vi "ProbeStationAutomation.vi"() -> ()   [LabVIEW 2020]
uses:
  Control 2.ctl
  C:/Users/User/Desktop/Automation/CurrentVersion/LabviewDXFViewer/bin/Release/LabviewDXFViewer.exe
  LabviewDXFViewer/bin/Release/LabviewDXFViewer.exe
  UIReferences.ctl
  WaferAlignmentType.ctl
  <vilib>/Utility/file.llb/Write Delimited Spreadsheet (DBL).vi
  Keithley 2600 Series/Keithley 2600 Series.lvlib
panel:
  in  "StartOxide":refnum<k24>(container)
  out "WaferAlignment":T1
  out "UiDefinition 3":T2
  in  "PathInfos":T3
  in  "UiDefinition 2":T2
  out "SweepInfo":T4
  out "error out":errorcluster
  out "Position 3":i32[](array[numeric])
  out "Position 2":i32[](array[numeric])
  out "Status":string="Please Load/Select probe site list"
  in  "Chip Orientation":i32(ring) items=["Horizontal", "Vertical"]
  in  "TextEditor":refnum<k24>(container)
  out "WaferTestPoints":string
  out "TestPointsLoaded":bool
  out "dxfFile":string
  out "error out 5":errorcluster
  out "Fit Array":string[][](array[string])
  out "error out 4":errorcluster
  out "error out 3":errorcluster
  out "Fit":dbl[][](array[numeric])
  out "IV Scan Data":dbl[][](array[numeric])
  out "Rotation Misalign":dbl[](array[numeric])
  out "Scale Misalign":dbl
  out "Position 1":i32[](array[numeric])
  in  "Microsites":refnum<k24>(container)
  in  "DXFCanvas":refnum<k24>(container)
  in  "WebCamViewer":refnum<k24>(container)
  in  "IV Curves":T5
  in  "Tab Control":T6(tab)
  in  "ClearPositions":bool
  in  "User":string
  in  "resetcontact":bool
  in  "EnableJoystick":bool
  in  "StartCycle":refnum<k24>(container)
  in  "Version":string
  in  "Experiment":string
  in  "Lower":refnum<k24>(container)
  in  "Raise":refnum<k24>(container)
  in  "West":refnum<k24>(container)
  in  "East":refnum<k24>(container)
  in  "North":refnum<k24>(container)
  in  "South":refnum<k24>(container)
  in  "Align Position 1":bool
  in  "Platten Move":refnum<k24>(container)
  in  "Masks":string(combo)
  in  "Move Position 1":bool
  in  "Align Position 3":bool
  in  "Position 3":bool
  in  "Align Position 2":bool
  in  "Position 2":bool
  in  "Die":string
  in  "Wafer":string
  in  "Jog (um) 2":dbl=100.0
  in  "Jog (um)":dbl=500.0
  in  "Load Mask":bool
  in  "Save Wafer":bool
  in  "Lift Distance (um)":dbl=2000.0
  in  "Quit":bool
  out "In Contact":bool
  out "Motor Position":string
  in  "Save Tag":string
  out "Capacitance":dbl
  in  "Current Range (A)":dbl=1e-10
  in  "Junction":string(combo)="None"
  in  "Sweeps":dbl=2.0
  in  "Number Points":dbl=200.0
  in  "Minimum (mV)":dbl=-100.0
  in  "Maxiumum (mV)":dbl=100.0
  in  "Source Measure Unit Channel (0: Channel A)":i32(ring) items=["Channel A", "Channel B"]
  in  "VISA resource name":refnum<visa-resource-name>="Keithley_2636A"
  in  "Scan":bool
  in  "Save Scan":bool
  out "Conductance":dbl
  out "Intercept":dbl
  out "XY Graph":cluster{"x":timestamp, "y":dbl}[](graph)
  in  "Steps Per micron":dbl=0.629
  in  "Stepper Controller Port":i32=3
  out "GetCameras":string[](array[string])
  in  "Wafer Definition File":path=path "C:/Users/User/Desktop/Automation/ASU FG Mask 21.08.26.dxf"
  in  "Wafer Units to microns":dbl=1.0
  in  "Data Path":path=path "C:/Data"
  # "Run Oxide"
  # "Optional Tags"
  # "Jog Platten"
  # "Platten Altitude"
  # "Run IVs"
  # "Cycle Step"
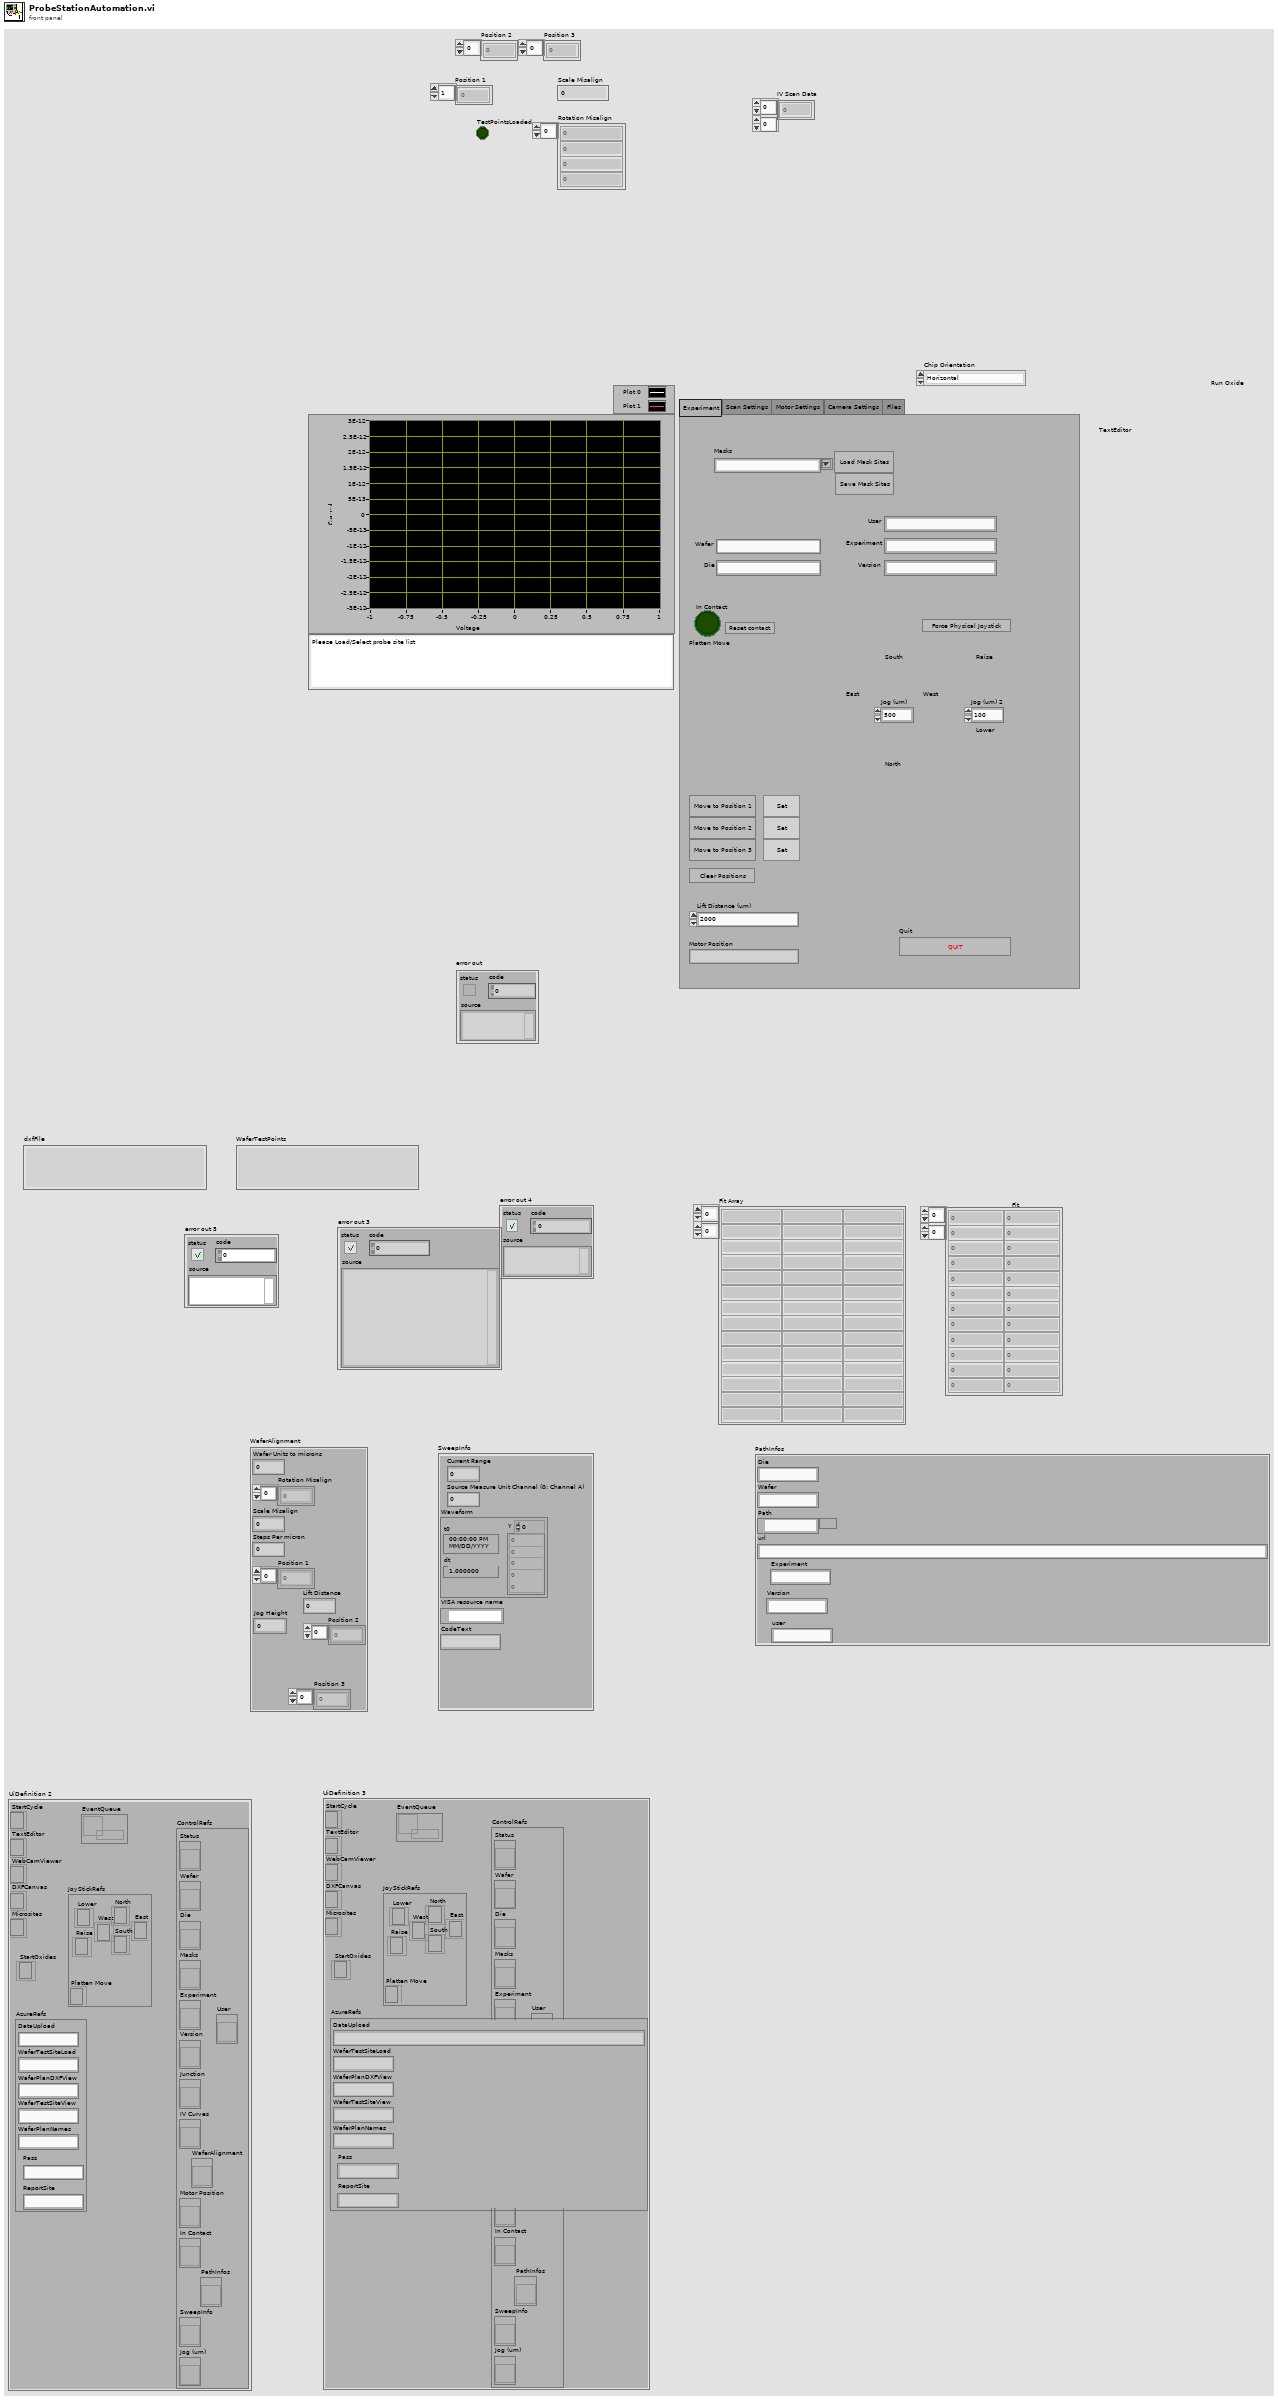
[diagram p1: front panel]
types:
  T1 = typedef "WaferAlignmentType.ctl" = cluster{"Wafer Units to microns":dbl, "Rotation Misalign":dbl[], "Scale Misalign":dbl, "Steps Per micron":dbl, "Position 1":i32[], "Position 2":i32[], "Lift Distance":i32, "Position 3":i32[], "Jog Height":i32}
  T2 = typedef "UIReferences.ctl" = cluster{"StartCycle":refnum<k24>, "TextEditor":refnum<k24>, "WebCamViewer":refnum<k24>, "DXFCanvas":refnum<k24>, "Microsites":refnum<k24>, "JoyStickRefs":cluster{"North":refnum<k24>, "Lower":refnum<k24>, "Raise":refnum<k24>, "Platten Move":refnum<k24>, "West":refnum<k24>, "East":refnum<k24>, "South":refnum<k24>}, "AzureRefs":cluster{"DataUpload":string, "WaferTestSiteLoad":string, "WaferPlanDXFView":string, "WaferTestSiteView":string, "WaferPlanNames":string, "Pass":string, "ReportSite":string}, "ControlRefs":cluster{"Status":refnum<vi>, "Wafer":refnum<vi>, "Die":refnum<vi>, "Masks":refnum<vi>, "Experiment":refnum<vi>, "Version":refnum<vi>, "Junction":refnum<vi>, "IV Curves":refnum<vi>, "Motor Position":refnum<vi>, "In Contact":refnum<vi>, "SweepInfo":refnum<vi>, "Jog (um)":refnum<vi>, "PathInfos":refnum<vi>, "User":refnum<vi>, "WaferAlignment":refnum<vi>}, "EventQueue":refnum<queue>, "StartOxides":refnum<k24>}
  T3 = cluster{"Die":string, "Wafer":string, "Path":path, "url":string, "Experiment":string, "Version":string, "user":string}
  T4 = cluster{"Current Range":dbl, "Source Measure Unit Channel (0: Channel A)":i32, "Waveform":waveform(dbl), "VISA resource name":refnum<visa-resource-name>, "CodeText":string}
  T5 = typedef "Control 2.ctl" = cluster{"Y":dbl[], "Current (A)":dbl[]}
  T6 = enum32{"Experiment", "Scan Settings", "Motor Settings", "Camera Settings", "Files"}
  T7 = cluster{"DataUpload":string, "WaferTestSiteLoad":string, "WaferPlanDXFView":string, "WaferTestSiteView":string, "WaferPlanNames":string, "Pass":string, "ReportSite":string}
  T8 = cluster{"North":refnum<k24>, "Lower":refnum<k24>, "Raise":refnum<k24>, "Platten Move":refnum<k24>, "West":refnum<k24>, "East":refnum<k24>, "South":refnum<k24>}
  T9 = cluster{"Status":refnum<vi>, "Wafer":refnum<vi>, "Die":refnum<vi>, "Masks":refnum<vi>, "Experiment":refnum<vi>, "Version":refnum<vi>, "Junction":refnum<vi>, "IV Curves":refnum<vi>, "Motor Position":refnum<vi>, "In Contact":refnum<vi>, "SweepInfo":refnum<vi>, "Jog (um)":refnum<vi>, "PathInfos":refnum<vi>, "User":refnum<vi>, "WaferAlignment":refnum<vi>}
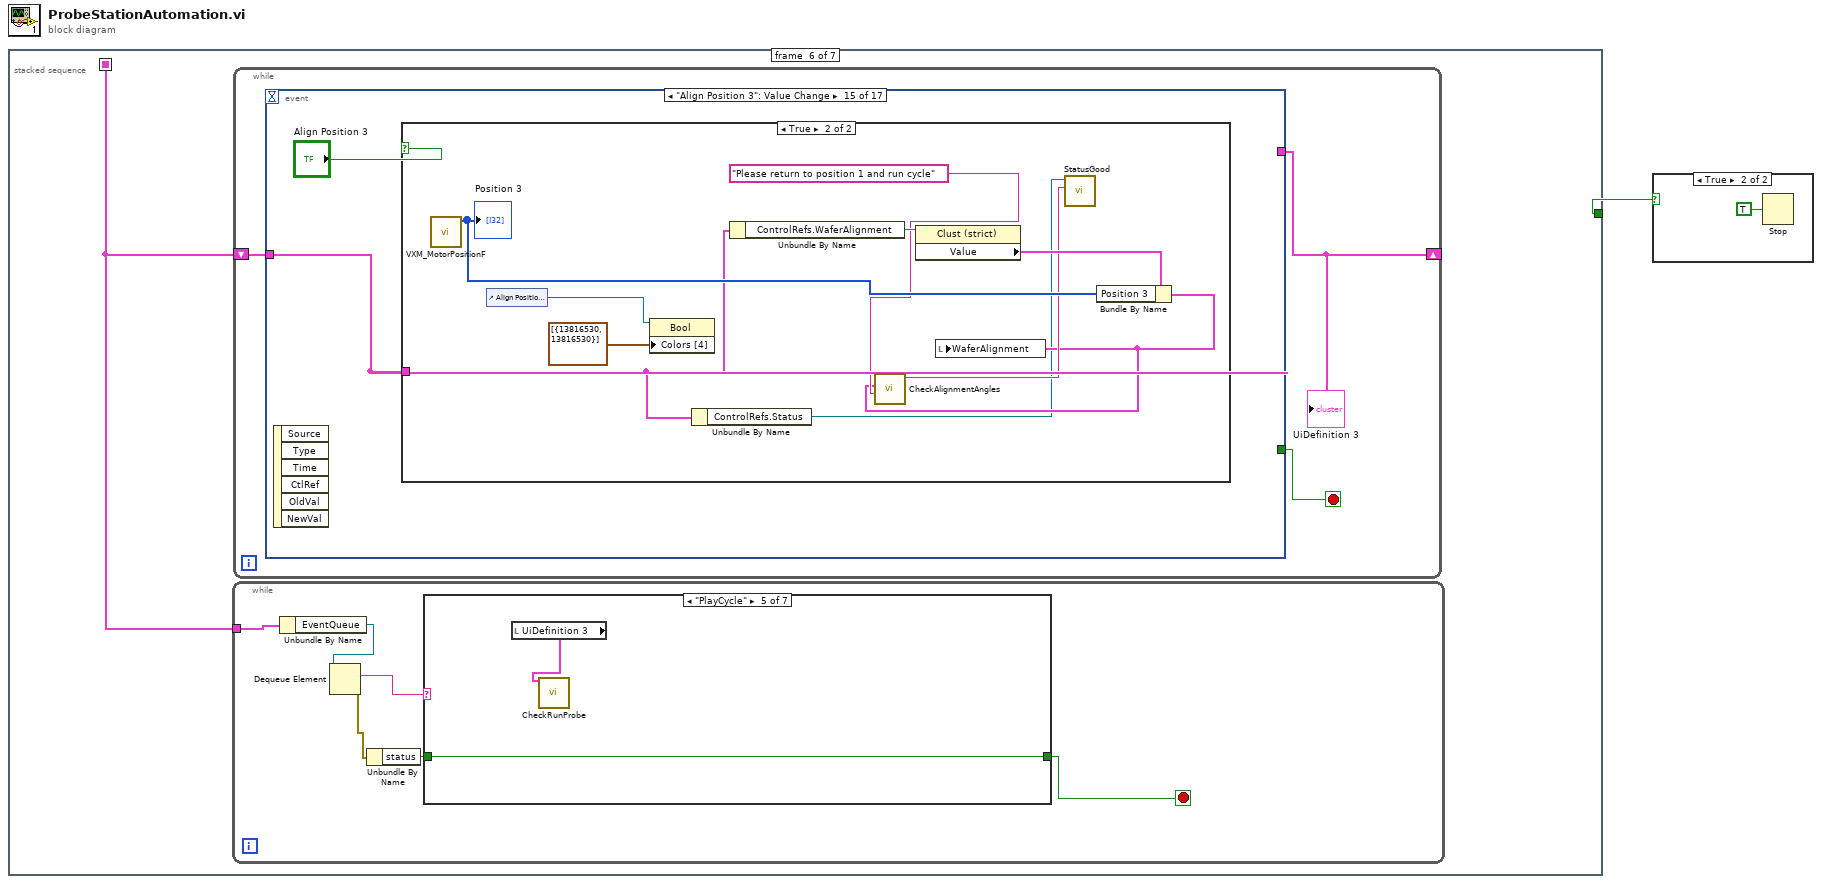
[diagram p0: block diagram]
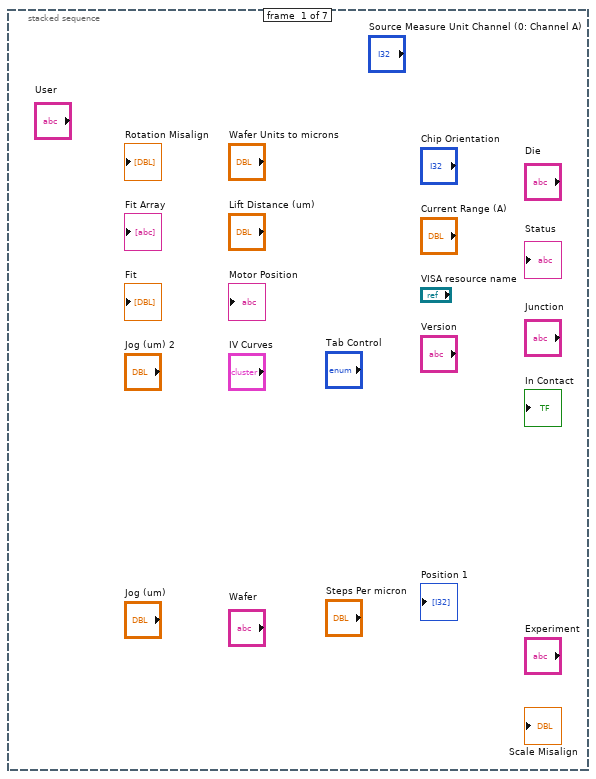
[diagram p3: hidden frame]
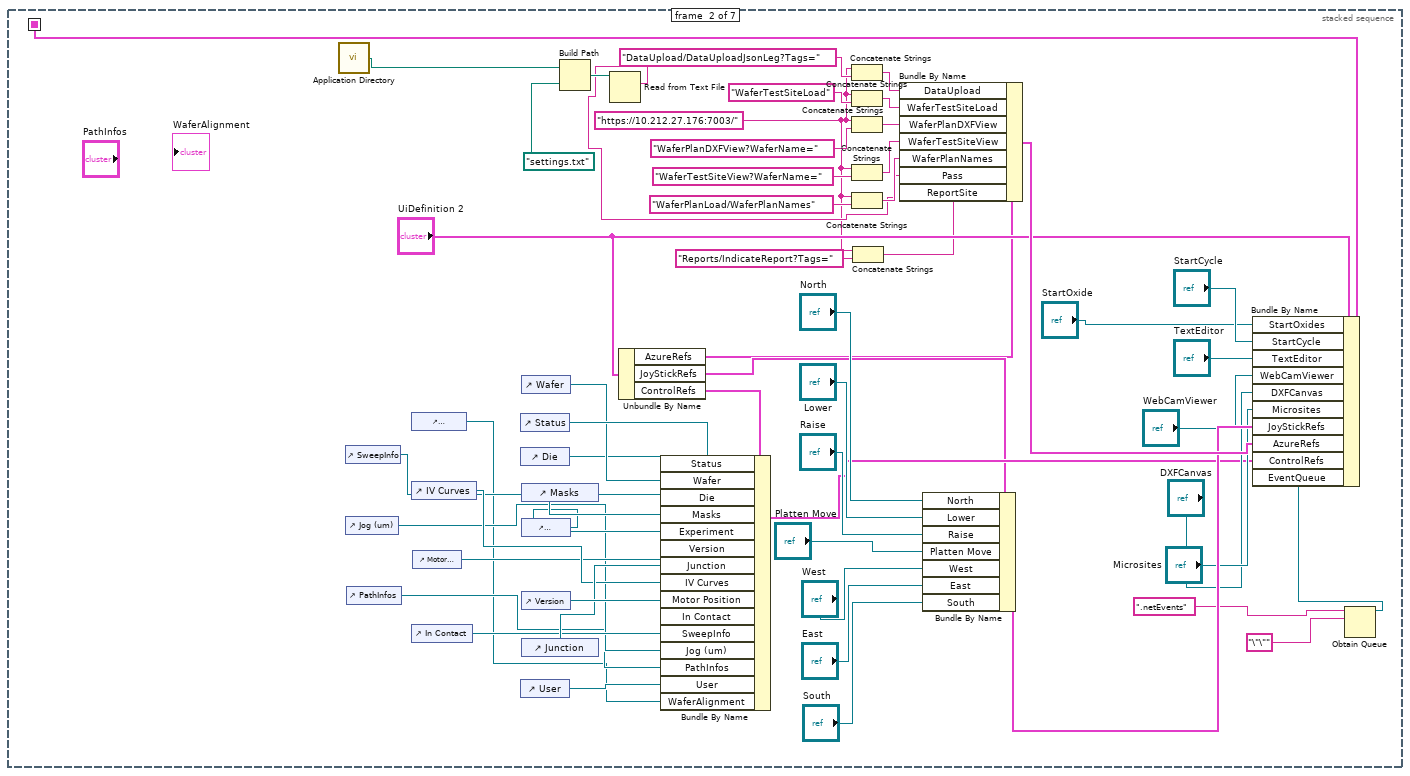
[diagram p4: hidden frame]
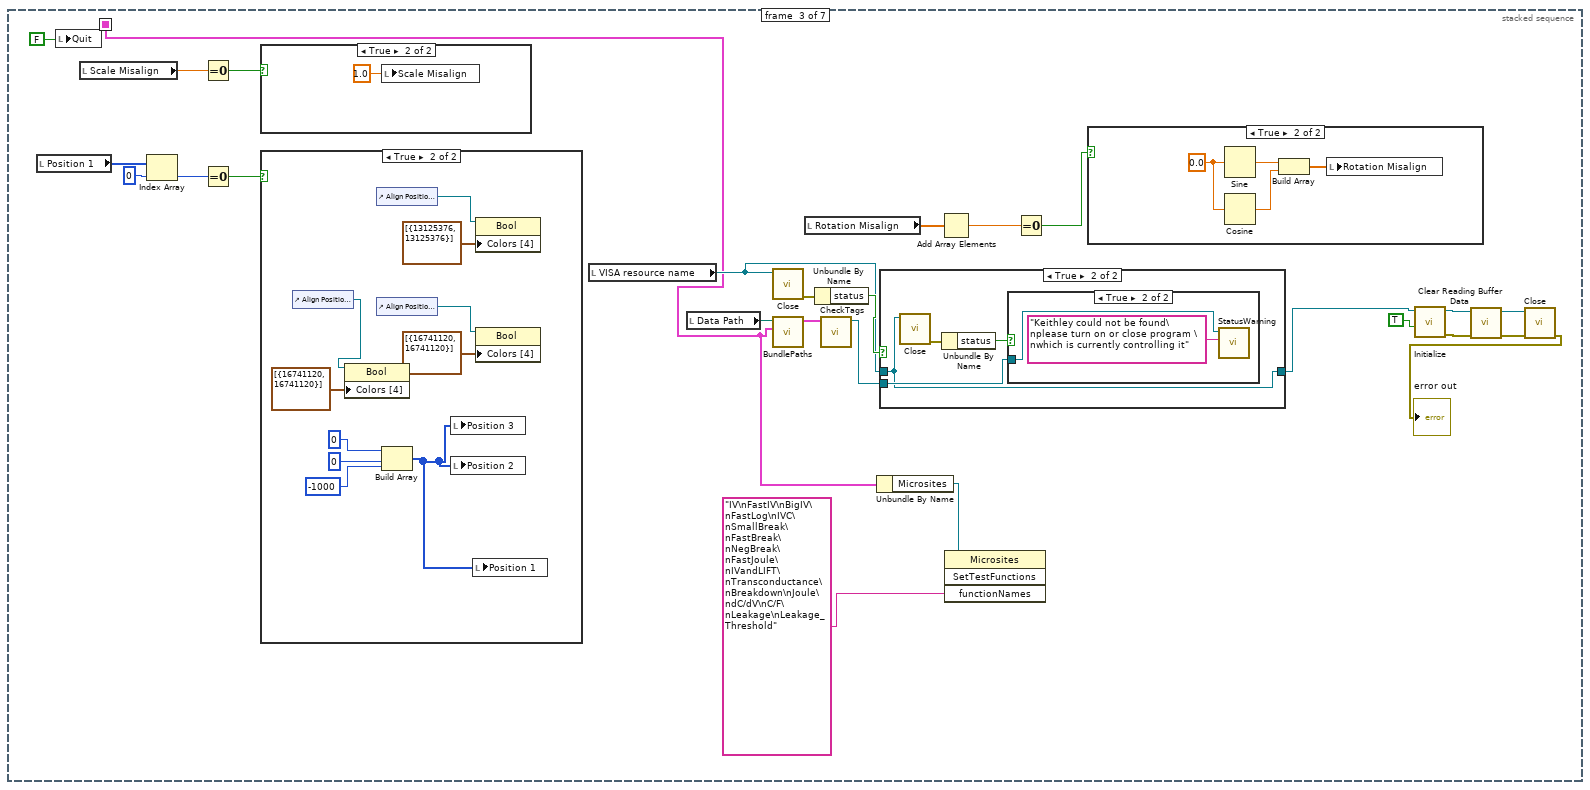
[diagram p5: hidden frame]
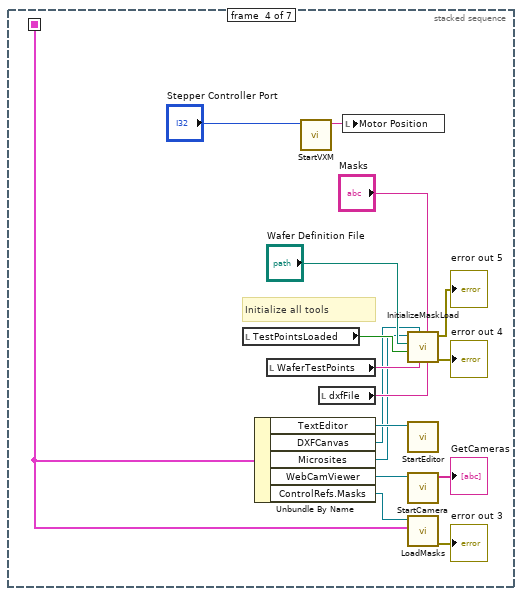
[diagram p11: hidden frame]
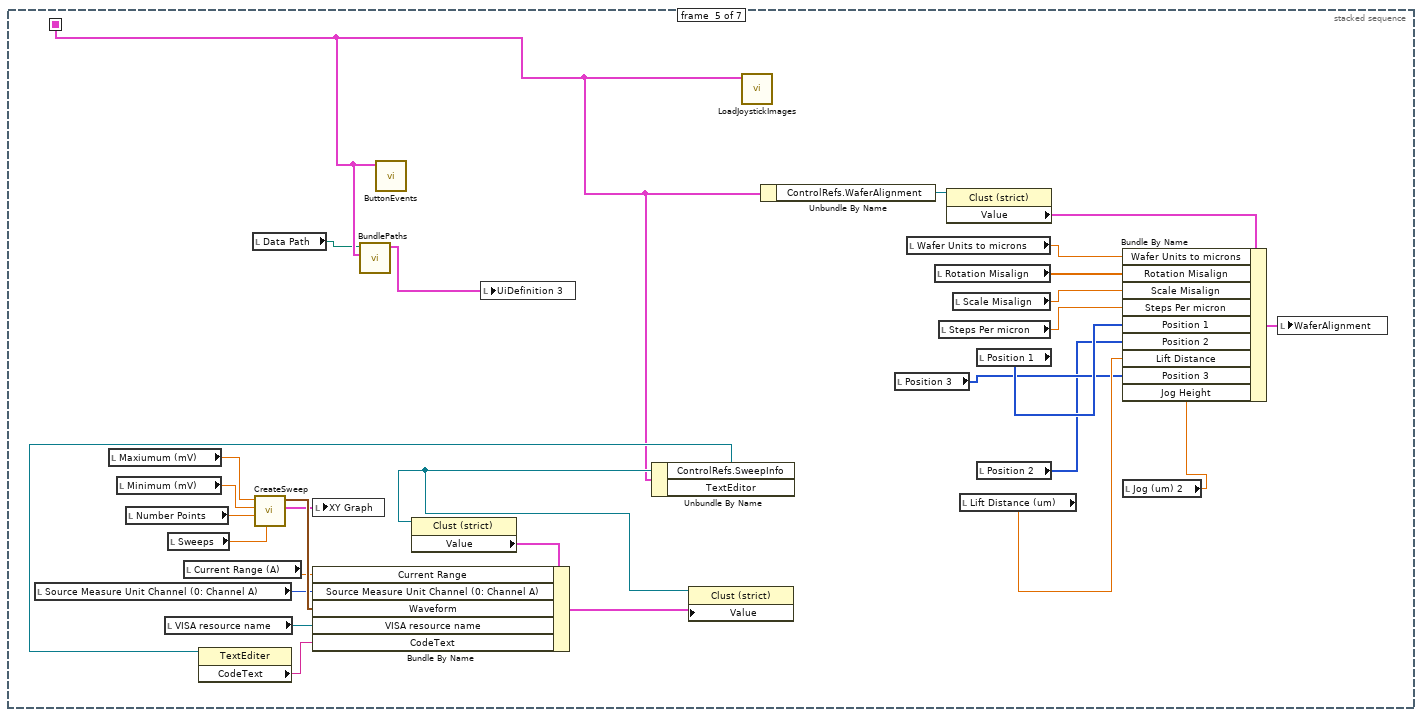
[diagram p12: hidden frame]
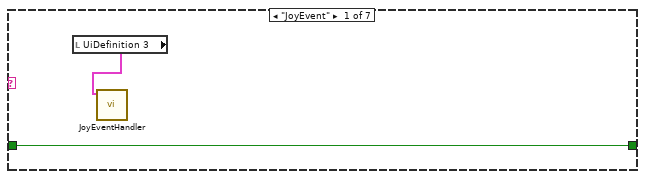
[diagram p13: hidden frame]
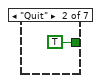
[diagram p14: hidden frame]
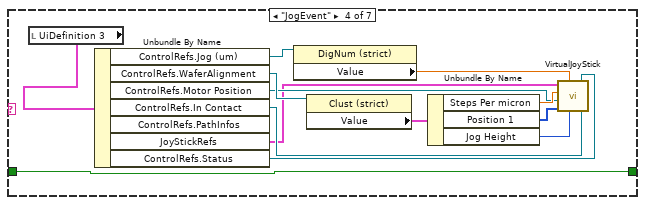
[diagram p16: hidden frame]
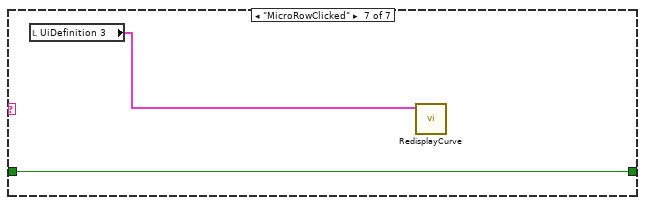
[diagram p18: hidden frame]
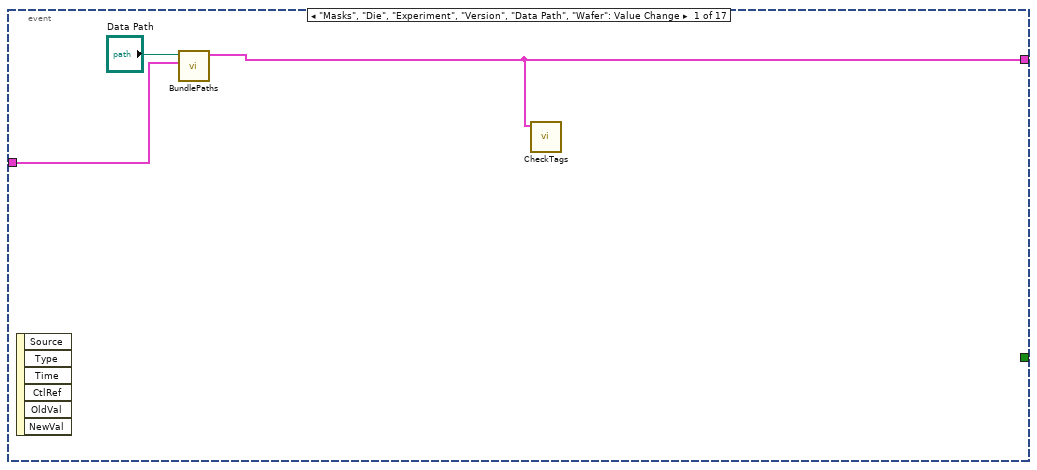
[diagram p19: hidden frame]
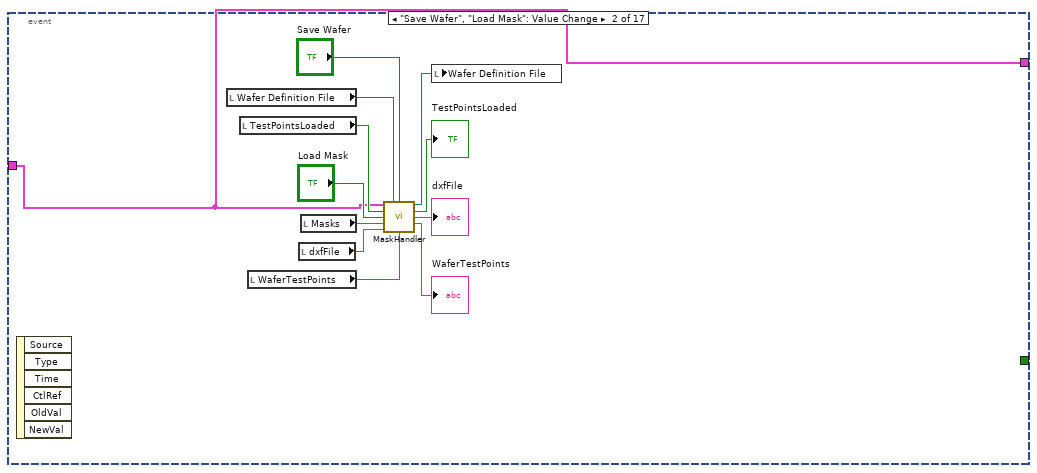
[diagram p20: hidden frame]
diagram:
  n1 = stacked-sequence {
    seq-local: [_ w44 _ _ _ _ _] -> [_ _ w60 w106 w125 w152 _]
    tunnel: [_ _ _ _ _ _ TRUE ("Quit")] -> w1
    frame #0 {
    }
    frame #1 {
      w4 = "https://10.212.27.176:7003/"
      n2 = call <vilib>:"Application Directory.vi"() -> ("Application Directory"=w2:path)
      n3 = control-ref of="SweepInfo"() -> (w29:refnum<vi>)
      n4 = control-ref of="Jog (um)"() -> (w28:refnum<vi>)
      n5 = control-ref of="PathInfos"() -> (w27:refnum<vi>)
      n6 = control-ref of="WaferAlignment"() -> (w6:refnum<vi>)
      n7 = control-ref of="IV Curves"() -> (w32:refnum<vi>)
      n8 = control-ref of="In Contact"() -> (w30:refnum<vi>)
      n9 = control-ref of="Motor Position"() -> (w31:refnum<vi>)
      n10 = control-ref of="Status"() -> (w39:refnum<vi>)
      n11 = control-ref of="Die"() -> (w37:refnum<vi>)
      n12 = control-ref of="User"() -> (w22:refnum<vi>)
      n13 = control-ref of="Wafer"() -> (w38:refnum<vi>)
      n14 = control-ref of="Masks"() -> (w36:refnum<vi>)
      n15 = control-ref of="Experiment"() -> (w35:refnum<vi>)
      n16 = control-ref of="Version"() -> (w34:refnum<vi>)
      n17 = control-ref of="Junction"() -> (w33:refnum<vi>)
      n18 = Build Path(base path=w2, name or relative path=path "settings.txt" ("file (use dialog)")) -> (appended path=w10:path)
      n19 = Read from Text File(file (use dialog)=w10) -> (text=w8:string)  [unwired: 3 in, 3 out]
      n20 = Unbundle By Name("UiDefinition 2") -> ("AzureRefs"=w21:T7, "JoyStickRefs"=w26:T8, "ControlRefs"=w41:T9)
      n21 = Bundle By Name(cluster=w41, "Status"=w39, "Wafer"=w38, "Die"=w37, "Masks"=w36, "Experiment"=w35, "Version"=w34, "Junction"=w33, "IV Curves"=w32, "Motor Position"=w31, "In Contact"=w30, "SweepInfo"=w29, "Jog (um)"=w28, "PathInfos"=w27, "User"=w22, "WaferAlignment"=w6) -> (w40:T9)
      n22 = Concatenate Strings(w4, "DataUpload/DataUploadJsonLeg?Tags=" ("url")) -> (w20:string)
      n23 = Concatenate Strings(w4, "WaferTestSiteLoad" ("url")) -> (w17:string)
      n24 = Concatenate Strings(w4, "WaferPlanDXFView?WaferName=" ("url")) -> (w15:string)
      n25 = Concatenate Strings(w4, "WaferTestSiteView?WaferName=" ("url")) -> (w13:string)
      n26 = Concatenate Strings(w4, "WaferPlanLoad/WaferPlanNames" ("url")) -> (w11:string)
      n27 = Concatenate Strings(w4, "Reports/IndicateReport?Tags=" ("string")) -> (w5:string)
      n28 = Bundle By Name(cluster=w21, "DataUpload"=w20, "WaferTestSiteLoad"=w17, "WaferPlanDXFView"=w15, "WaferTestSiteView"=w13, "WaferPlanNames"=w11, "Pass"=w8, "ReportSite"=w5) -> (w57:T7)
      n29 = Bundle By Name(cluster=w26, "North"="North", "Lower"="Lower", "Raise"="Raise", "Platten Move"="Platten Move", "West"="West", "East"="East", "South"="South") -> (w53:T8)
      n30 = Obtain Queue(name (unnamed)=".netEvents", element data type="\"\"") -> (queue out=w23:refnum<queue>)  [unwired: 3 in, 2 out]
      n31 = Bundle By Name(cluster="UiDefinition 2", "StartOxides"="StartOxide", "StartCycle"="StartCycle", "TextEditor"="TextEditor", "WebCamViewer"="WebCamViewer", "DXFCanvas"="DXFCanvas", "Microsites"="Microsites", "JoyStickRefs"=w53, "AzureRefs"=w57, "ControlRefs"=w40, "EventQueue"=w23) -> (w44:T2)
    }
    frame #2 {
      n32 = local read "Position 1"() -> (w82:i32[])
      n33 = local write "Quit"(FALSE) -> ()
      n34 = local read "Scale Misalign"() -> (w77:dbl)
      n35 = Index Array(array=w82, index=0) -> (element=w83:i32)
      n36 = Equal To 0?(x=w77) -> (x = 0?=w76:bool)
      n37 = Equal To 0?(x=w83) -> (x = 0?=w81:bool)
      n38 = case shown="True" w76 {
        frame False {
        }
        frame True {
          n39 = local write "Scale Misalign"(1.0 ("Scale Misalign")) -> ()
        }
      }
      n40 = case shown="True" w81 {
        frame False {
        }
        frame True {
          n41 = control-ref of="Align Position 3"() -> (w91:refnum<vi>)
          n42 = property class="Bool"(reference=w91, "Colors [4]"=cluster{u32, u32}[] [{16741120, 16741120}]) -> ()  [unwired: 1 in, 2 out]
          n43 = control-ref of="Align Position 1"() -> (w100:refnum<vi>)
          n44 = control-ref of="Align Position 2"() -> (w98:refnum<vi>)
          n45 = Build Array(0 ("Y"), 0 ("X"), -1000) -> (w93:i32[])
          n46 = local write "Position 3"(w93) -> ()
          n47 = local write "Position 2"(w93) -> ()
          n48 = local write "Position 1"(w93) -> ()
          n49 = property class="Bool"(reference=w100, "Colors [4]"=cluster{u32, u32}[] [{13125376, 13125376}]) -> ()  [unwired: 1 in, 2 out]
          n50 = property class="Bool"(reference=w98, "Colors [4]"=cluster{u32, u32}[] [{16741120, 16741120}]) -> ()  [unwired: 1 in, 2 out]
        }
      }
      n51 = local read "VISA resource name"() -> (w69:refnum<visa-resource-name>)
      n52 = local read "Data Path"() -> (w66:path)
      n53 = call "Close.vi"("VISA resource name"=w69) -> ("error out"=w73:errorcluster)  [unwired: 10 in]
      n54 = call "BundlePaths.vi"("Data Path"=w66, "UiDefinition 2"=w60) -> ("UiDefinition 3"=w67:T2)  [unwired: 8 in]
      n55 = local read "Rotation Misalign"() -> (w80:dbl[])
      n56 = Unbundle By Name(w73) -> ("status"=w72:bool)
      n57 = call "CheckTags.vi"("UiDefinition 2"=w67) -> ("StatusOut"=w71:refnum<vi>)  [unwired: 10 in]
      n58 = Unbundle By Name(w60) -> ("Microsites"=w59:refnum<k24>)
      n59 = case shown="True" w72 {
        tunnel: w71 -> [_ w88]
        tunnel: w69 -> [w84 w87]
        tunnel: [w84 w87] -> w68
        frame False {
        }
        frame True {
          n60 = call "Close.vi"("VISA resource name"=w87) -> ("error out"=w86:errorcluster)  [unwired: 10 in]
          n61 = Unbundle By Name(w86) -> ("status"=w85:bool)
          n62 = case shown="True" w85 {
            tunnel: w88 -> [_ w89]
            frame False {
            }
            frame True {
              n63 = call "StatusWarning.vi"("Text.Text"="Keithley could not be found\nplease turn on or close program \nwhich is currently controlling it", "String in"=w89) -> ()  [unwired: 10 in]
            }
          }
        }
      }
      n64 = Add Array Elements(numeric array=w80) -> (sum=w79:dbl)
      n65 = invoke class="Microsites" method="SetTestFunctions"(reference=w59, "functionNames"="IV\nFastIV\nBigIV\nFastLog\nIVC\nSmallBreak\nFastBreak\nNegBreak\nFastJoule\nIVandLIFT\nTransconductance\nBreakdown\nJoule\ndC/dV\nC/F\nLeakage\nLeakage_Threshold") -> ()  [unwired: 2 in, 4 out]
      n66 = Equal To 0?(x=w79) -> (x = 0?=w78:bool)
      n67 = case shown="True" w78 {
        frame False {
        }
        frame True {
          w101 = 0.0 ("x")
          n68 = Sine(x=w101) -> (sin(x)=w104:dbl)
          n69 = Cosine(x=w101) -> (cos(x)=w103:dbl)
          n70 = Build Array(w104, w103) -> (w102:dbl[])
          n71 = local write "Rotation Misalign"(w102) -> ()
        }
      }
      n72 = call "Initialize.vi"("Reset (True)"=TRUE, "VISA resource name"=w68) -> ("error out"=w64:errorcluster, "VISA resource name out"=w65:refnum<visa-resource-name>)  [unwired: 8 in]
      n73 = call "Clear Reading Buffer Data.vi"("error in (no error)"=w64, "VISA resource name"=w65) -> ("error out"=w63:errorcluster, "VISA resource name out"=w62:refnum<visa-resource-name>)  [unwired: 8 in]
      n74 = call "Close.vi"("error in (no error)"=w63, "VISA resource name"=w62) -> ("error out"=→"error out":errorcluster)  [unwired: 9 in]
    }
    frame #3 {
      # "Initialize all tools"
      n75 = local read "TestPointsLoaded"() -> (w117:bool)
      n76 = Unbundle By Name(w106) -> ("TextEditor"=w111:refnum<k24>, "DXFCanvas"=w110:refnum<k24>, "Microsites"=w109:refnum<k24>, "WebCamViewer"=w108:refnum<k24>, "ControlRefs.Masks"=w107:refnum<vi>)
      n77 = local read "WaferTestPoints"() -> (w116:string)
      n78 = call "StartVXM.vi"("Stepper Controller Port"="Stepper Controller Port") -> ("String"=w112:string)  [unwired: 10 in]
      n79 = local read "dxfFile"() -> (w115:string)
      n80 = local write "Motor Position"(w112) -> ()
      n81 = call "InitializeMaskLoad.vi"("dxfFile"=w115, "Masks"="Masks", "WaferTestPoints"=w116, "DXFCanvas"=w110, "TestPointsLoaded"=w117, "Wafer Definition File"="Wafer Definition File", "MicrositesRef"=w109) -> ("error out"=→"error out 4":errorcluster, "error out 5"=→"error out 5":errorcluster)  [unwired: 3 in]
      n82 = call "StartEditor.vi"("CodeEditorRef"=w111) -> ()  [unwired: 11 in]
      n83 = call "StartCamera.vi"("WebCamViewerRef"=w108) -> ("GetCameras"=→"GetCameras":string[])  [unwired: 10 in]
      n84 = call "LoadMasks.vi"("UiDefinition 2"=w106, "ComboBox in"=w107) -> ("error out"=→"error out 3":errorcluster)  [unwired: 9 in]
    }
    frame #4 {
      n85 = local read "Source Measure Unit Channel (0: Channel A)"() -> (w134:i32)
      n86 = local read "Maxiumum (mV)"() -> (w131:dbl)
      n87 = local read "Minimum (mV)"() -> (w130:dbl)
      n88 = local read "Number Points"() -> (w129:dbl)
      n89 = local read "VISA resource name"() -> (w139:refnum<visa-resource-name>)
      n90 = local read "Sweeps"() -> (w128:dbl)
      n91 = local read "Current Range (A)"() -> (w133:dbl)
      n92 = local read "Data Path"() -> (w123:path)
      n93 = call "CreateSweep.vi"("Sweeps"=w128, "Number Points"=w129, "Minimum Voltage"=w130, "Maxiumum Voltage"=w131) -> ("XY pairs"=w127:cluster{"x":timestamp, "y":dbl}[], "Waveform"=w135:waveform(dbl))  [unwired: 6 in]
      n94 = local write "XY Graph"(w127) -> ()
      n95 = call "BundlePaths.vi"("Data Path"=w123, "UiDefinition 2"=w125) -> ("UiDefinition 3"=w124:T2)  [unwired: 8 in]
      n96 = call "ButtonEvents.vi"("UiDefinition"=w125) -> ()  [unwired: 11 in]
      n97 = local write "UiDefinition 3"(w124) -> ()
      n98 = Unbundle By Name(w125) -> ("ControlRefs.SweepInfo"=w137:refnum<vi>, "TextEditor"=w138:refnum<k24>)
      n99 = property class="TextEditer"(reference=w138) -> ("CodeText"=w140:string)  [unwired: 1 in, 2 out]
      n100 = property class="Clust (strict)"(reference=w137) -> ("Value"=w136:T4)  [unwired: 1 in, 2 out]
      n101 = Bundle By Name(cluster=w136, "Current Range"=w133, "Source Measure Unit Channel (0: Channel A)"=w134, "Waveform"=w135, "VISA resource name"=w139, "CodeText"=w140) -> (w132:T4)
      n102 = property class="Clust (strict)"(reference=w137, "Value"=w132) -> ()  [unwired: 1 in, 2 out]
      n103 = call "LoadJoystickImages.vi"("UiDefinition 2"=w125) -> ()  [unwired: 11 in]
      n104 = Unbundle By Name(w125) -> ("ControlRefs.WaferAlignment"=w151:refnum<vi>)
      n105 = local read "Position 3"() -> (w143:i32[])
      n106 = local read "Wafer Units to microns"() -> (w148:dbl)
      n107 = local read "Rotation Misalign"() -> (w147:dbl[])
      n108 = local read "Steps Per micron"() -> (w141:dbl)
      n109 = property class="Clust (strict)"(reference=w151) -> ("Value"=w150:T1)  [unwired: 1 in, 2 out]
      n110 = local read "Scale Misalign"() -> (w146:dbl)
      n111 = local read "Lift Distance (um)"() -> (w144:dbl)
      n112 = local read "Position 1"() -> (w145:i32[])
      n113 = local read "Position 2"() -> (w142:i32[])
      n114 = local read "Jog (um) 2"() -> (w126:dbl)
      n115 = Bundle By Name(cluster=w150, "Wafer Units to microns"=w148, "Rotation Misalign"=w147, "Scale Misalign"=w146, "Steps Per micron"=w141, "Position 1"=w145, "Position 2"=w142, "Lift Distance"=w144, "Position 3"=w143, "Jog Height"=w126) -> (w149:T1)
      n116 = local write "WaferAlignment"(w149) -> ()
    }
    frame #5 {
      n117 = while {
        tunnel: w152 -> [w153]
        stop <- w154 stop-if-true
        n118 = Unbundle By Name(w153) -> ("EventQueue"=w157:refnum<queue>)
        n119 = Dequeue Element(queue=w157) -> (element=w158:string, error out=w156:errorcluster)  [unwired: 2 in, 2 out]
        n120 = Unbundle By Name(w156) -> ("status"=w155:bool)
        n121 = case shown="\"PlayCycle\"" w158 {
          tunnel: w155 -> [w160 _ w162 w164 w177 w178 w180]
          tunnel: [w160 TRUE ("status") w162 w164 w177 w178 w180] -> w154
          frame "JoyEvent" {
            n122 = local read "UiDefinition 3"() -> (w159:T2)
            n123 = call "JoyEventHandler.vi"("UiDefinition"=w159) -> ()  [unwired: 11 in]
          }
          frame "Quit" {
          }
          frame Default {
          }
          frame "JogEvent" {
            n124 = local read "UiDefinition 3"() -> (w163:T2)
            n125 = Unbundle By Name(w163) -> ("ControlRefs.Jog (um)"=w167:refnum<vi>, "ControlRefs.WaferAlignment"=w175:refnum<vi>, "ControlRefs.Motor Position"=w172:refnum<vi>, "ControlRefs.In Contact"=w170:refnum<vi>, "JoyStickRefs"=w168:T8, "ControlRefs.Status"=w165:refnum<vi>)  [unwired: 1 out]
            n126 = property class="DigNum (strict)"(reference=w167) -> ("Value"=w166:dbl)  [unwired: 1 in, 2 out]
            n127 = property class="Clust (strict)"(reference=w175) -> ("Value"=w174:T1)  [unwired: 1 in, 2 out]
            n128 = Unbundle By Name(w174) -> ("Steps Per micron"=w173:dbl, "Position 1"=w171:i32[], "Jog Height"=w169:i32)
            n129 = call "VirtualJoyStick.vi"("In Contact"=w170, "Status"=w165, "Jog (um) raise"=w169, "Jog (um)"=w166, "Position 1"=w171, "Motor Zero"=w172, "Steps Per micron"=w173, "JoyStickRefs"=w168) -> ()
          }
          frame "PlayCycle" {
            n130 = local read "UiDefinition 3"() -> (w176:T2)
            n131 = call "CheckRunProbe.vi"("UiDefinition"=w176) -> ()  [unwired: 15 in]
          }
          frame "OxideCycle" {
          }
          frame "MicroRowClicked" {
            n132 = local read "UiDefinition 3"() -> (w179:T2)
            n133 = call "RedisplayCurve.vi"("UiDefinition 3"=w179) -> ()  [unwired: 11 in]
          }
        }
      }
      n134 = while {
        shift-right: [w182] -> _
        shift-left: w152 -> [w183]
        stop <- w181 stop-if-true
        n135 = event shown="[14] \"Align Position 3\": Value Change" {
          selector: _ -> [_ _ _ _ _ _ _ _ _ _ _ _ _ _ _ _ _]
          dyn-events: _ -> [_ _ _ _ _ _ _ _ _ _ _ _ _ _ _ _ _]
          timeout: _ -> [_ _ _ _ _ _ _ _ _ _ _ _ _ _ _ _ _]
          tunnel: w183 -> [w185 w187 w199 w206 w224 w230 w239 w248 w256 w260 w264 w328 w330 w346 w350 w362 w375]
          tunnel: [w184 w187 w199 w206 w224 w230 w239 w248 w256 w260 w264 w328 w330 w346 w350 w362 w375] -> w182
          tunnel: [_ _ _ _ _ _ "Quit" _ _ _ _ _ _ _ _ _ _] -> w181
          event "Masks", "Die", "Experiment", "Version", "Data Path", "Wafer": Value Change {
            n136 = event-data() -> ()  [unwired: 1 in, 6 out]
            n137 = call "BundlePaths.vi"("Data Path"="Data Path", "UiDefinition 2"=w185) -> ("UiDefinition 3"=w184:T2)  [unwired: 8 in]
            n138 = call "CheckTags.vi"("UiDefinition 2"=w184) -> ()  [unwired: 10 in, 1 out]
          }
          event "Save Wafer", "Load Mask": Value Change {
            n139 = event-data() -> ()  [unwired: 1 in, 6 out]
            n140 = local read "Wafer Definition File"() -> (w195:path)
            n141 = local read "TestPointsLoaded"() -> (w192:bool)
            n142 = local read "WaferTestPoints"() -> (w196:string)
            n143 = local read "dxfFile"() -> (w198:string)
            n144 = local read "Masks"() -> (w189:string)
            n145 = call "MaskHandler.vi"("UiDefinition 2"=w187, "Wafer Definition File"=w195, "Save Wafer"="Save Wafer", "TestPointsLoaded in"=w192, "Load Mask"="Load Mask", "Masks"=w189, "dxfFile"=w198, "WaferTestPoints"=w196) -> ("Path"=w193:path, "TestPointsLoaded out"=→"TestPointsLoaded":bool, "body 2"=→"dxfFile":string, "body"=→"WaferTestPoints":string)  [unwired: 4 in]
            n146 = local write "Wafer Definition File"(w193) -> ()
          }
          event "Scan": Value Change {
            # "On request IV curve"
            n147 = event-data() -> ()  [unwired: 1 in, 6 out]
            n148 = case shown="True" "Scan" {
              tunnel: w199 -> [_ w202]
              frame False {
              }
              frame True {
                n149 = call "SingleIV.vi"("UiDefinition 2"=w202) -> ("appended array"=→"IV Scan Data":dbl[][], "CapacitanceIV"=→"Capacitance":dbl, "slope"=→"Conductance":dbl, "intercept"=→"Intercept":dbl)  [unwired: 11 in]
              }
            }
          }
          event "Align Position 1": Value Change {
            n150 = event-data() -> ()  [unwired: 1 in, 6 out]
            n151 = Unbundle By Name(w206) -> ("ControlRefs.Status"=w207:refnum<vi>)
            n152 = case shown="True" "Align Position 1" {
              tunnel: w207 -> [_ w216]
              tunnel: w206 -> [_ w214]
              frame False {
              }
              frame True {
                n153 = Unbundle By Name(w214) -> ("ControlRefs.WaferAlignment"=w215:refnum<vi>)
                n154 = control-ref of="Align Position 1"() -> (w219:refnum<vi>)
                n155 = local write "In Contact"(TRUE) -> ()
                n156 = property class="Bool"(reference=w219, "Colors [4]"=cluster{u32, u32}[] [{13816530, 13816530}]) -> ()  [unwired: 1 in, 2 out]
                n157 = property class="Clust (strict)"(reference=w215) -> ("Value"=w213:T1)  [unwired: 1 in, 2 out]
                n158 = call "VXM_MotorPositionF.vi"() -> ("Position"=w212:i32[])  [unwired: 11 in]
                n159 = Bundle By Name(cluster=w213, "Position 1"=w212) -> (w209:T1)
                n160 = local write "Position 1"(w212) -> ()
                n161 = call "CheckAlignmentAngles.vi"("Status in"="Align Position 2 or run cycle" ("Status"), "Value"=w209) -> ("Status out"=w210:string)  [unwired: 9 in]
                n162 = call "StatusGood.vi"("Text.Text"=w210, "String in"=w216) -> ()  [unwired: 10 in]
                n163 = local write "WaferAlignment"(w209) -> ()
              }
            }
          }
          event "Minimum (mV)", "Maxiumum (mV)", "Number Points", "Sweeps": Value Change {
            n164 = event-data() -> ()  [unwired: 1 in, 6 out]
            n165 = Unbundle By Name(w224) -> ("ControlRefs.SweepInfo"=w220:refnum<vi>)
            n166 = call "CreateSweep.vi"("Sweeps"="Sweeps", "Number Points"="Number Points", "Minimum Voltage"="Minimum (mV)", "Maxiumum Voltage"="Maxiumum (mV)") -> ("XY pairs"=→"XY Graph":cluster{"x":timestamp, "y":dbl}[], "Waveform"=w222:waveform(dbl))  [unwired: 6 in]
            n167 = property class="Clust (strict)"(reference=w220) -> ("Value"=w223:T4)  [unwired: 1 in, 2 out]
            n168 = Bundle By Name(cluster=w223, "Waveform"=w222) -> (w221:T4)
            n169 = property class="Clust (strict)"(reference=w220, "Value"=w221) -> ()  [unwired: 1 in, 2 out]
          }
          event "Current Range (A)", "VISA resource name", "Source Measure Unit Channel (0: Channel A)": Value Change {
            n170 = event-data() -> ()  [unwired: 1 in, 6 out]
            n171 = Unbundle By Name(w230) -> ("ControlRefs.SweepInfo"=w233:refnum<vi>, "TextEditor"=w234:refnum<k24>)
            n172 = local read "Source Measure Unit Channel (0: Channel A)"() -> (w235:i32)
            n173 = local read "VISA resource name"() -> (w236:refnum<visa-resource-name>)
            n174 = local read "Current Range (A)"() -> (w237:dbl)
            n175 = property class="Clust (strict)"(reference=w233) -> ("Value"=w231:T4)  [unwired: 1 in, 2 out]
            n176 = property class="TextEditer"(reference=w234) -> ("CodeText"=w238:string)  [unwired: 1 in, 2 out]
            n177 = Bundle By Name(cluster=w231, "Current Range"=w237, "Source Measure Unit Channel (0: Channel A)"=w235, "VISA resource name"=w236, "CodeText"=w238) -> (→"SweepInfo":T4)
          }
          event "Quit": Value Change {
            n178 = event-data() -> ()  [unwired: 1 in, 6 out]
            n179 = Unbundle By Name(w239) -> ("EventQueue"=w241:refnum<queue>)
            n180 = Enqueue Element(queue=w241, element="Quit") -> ()  [unwired: 2 in, 3 out]
          }
          event "Position 1", "Wafer Units to microns", "Rotation Misalign", "Scale Misalign", "Steps Per micron", "Lift Distance (um)", "Jog (um) 2": Value Change {
            n181 = event-data() -> ()  [unwired: 1 in, 6 out]
            n182 = Unbundle By Name(w248) -> ("ControlRefs.WaferAlignment"=w250:refnum<vi>)
            n183 = property class="Clust (strict)"(reference=w250) -> ("Value"=w249:T1)  [unwired: 1 in, 2 out]
            n184 = local read "Wafer Units to microns"() -> (w254:dbl)
            n185 = local read "Rotation Misalign"() -> (w251:dbl[])
            n186 = local read "Lift Distance (um)"() -> (w245:dbl)
            n187 = local read "Steps Per micron"() -> (w252:dbl)
            n188 = local read "Scale Misalign"() -> (w253:dbl)
            n189 = local read "Jog (um) 2"() -> (w244:dbl)
            n190 = local read "Position 1"() -> (w255:i32[])
            n191 = local read "Position 2"() -> (w247:i32[])
            n192 = local read "Position 3"() -> (w246:i32[])
            n193 = Bundle By Name(cluster=w249, "Wafer Units to microns"=w254, "Rotation Misalign"=w251, "Scale Misalign"=w253, "Steps Per micron"=w252, "Position 1"=w255, "Position 2"=w247, "Lift Distance"=w245, "Position 3"=w246, "Jog Height"=w244) -> (w243:T1)
            n194 = local write "WaferAlignment"(w243) -> ()
          }
          event "Move Position 1": Value Change {
            n195 = event-data() -> ()  [unwired: 1 in, 6 out]
            n196 = local read "In Contact"() -> (w259:bool)
            n197 = call "MovePos1.vi"("In Contact in"=w259, "Move Position 1"="Move Position 1", "UiDefinition 2"=w256) -> ("In Contact out"=w258:bool)  [unwired: 8 in]
            n198 = local write "In Contact"(w258) -> ()
          }
          event "Position 2": Value Change {
            n199 = event-data() -> ()  [unwired: 1 in, 6 out]
            n200 = local read "In Contact"() -> (w263:bool)
            n201 = call "MoveToPosition2.vi"("In Contact in"=w263, "Position in"="Position 2", "UiDefinition 2"=w260) -> ("In Contact out"=w262:bool)  [unwired: 8 in]
            n202 = local write "In Contact"(w262) -> ()
          }
          event "Save Scan": Value Change {
            n203 = event-data() -> ()  [unwired: 1 in, 6 out]
            n204 = case shown="True" "Save Scan" {
              tunnel: w264 -> [_ w272]
              frame False {
              }
              frame True {
                n205 = Unbundle By Name(w272) -> ("ControlRefs.PathInfos"=w275:refnum<vi>)  [unwired: 1 out]
                n206 = local read "Junction"() -> (w269:string)
                n207 = property class="Clust (strict)"(reference=w275) -> ("Value"=w274:T3)  [unwired: 1 in, 2 out]
                n208 = Not Equal?(x="None", y=w269) -> (x != y?=w271:bool)
                n209 = local read "IV Scan Data"() -> (w278:dbl[][])
                n210 = Unbundle By Name(w274) -> ("Path"=w267:path, "url"=w273:string)
                n211 = call <vilib>:"Check if File or Folder Exists.vi"("path"=w267) -> ("file or folder exists?"=w268:bool)  [unwired: 8 in, 2 out]
                n212 = case shown="False" w268 {
                  tunnel: w267 -> [w280 w281]
                  tunnel: [w279 w281] -> w266
                  frame False {
                    n213 = Create Folder(path (use dialog)=w280) -> (created path=w279:path)  [unwired: 2 in, 2 out]
                  }
                  frame True {
                  }
                }
                n214 = case shown="True" TRUE {
                  tunnel: w278 -> [_ w290]
                  tunnel: "Save Tag" -> [_ w284]
                  tunnel: w271 -> [_ w286]
                  tunnel: w269 -> [_ w283]
                  tunnel: w266 -> [_ w282]
                  frame False {
                  }
                  frame True {
                    n215 = Empty String/Path?(string/path=w284) -> (empty?=w285:bool)
                    n216 = case shown="True" w286 {
                      tunnel: [w294 FALSE ("cancelled")] -> w289
                      tunnel: [w293 w295] -> w288
                      tunnel: [w292 errorcluster {"status"=FALSE, "code"=0, "source"=""} ("error out")] -> w287
                      tunnel: w285 -> [_ w299]
                      tunnel: w282 -> [w291 w298]
                      tunnel: w284 -> [_ w297]
                      tunnel: w283 -> [_ w296]
                      frame False {
                        n217 = call "File Dialog"("start path"=w291) -> ("selected path"=w293:path, "cancelled"=w294:bool, "error out"=w292:errorcluster)  [unwired: 11 in, 1 out]
                      }
                      frame True {
                        n218 = case shown="True" w299 {
                          tunnel: w298 -> [w308 w312]
                          tunnel: [w307 w313] -> w295
                          tunnel: w297 -> [w303 _]
                          tunnel: w296 -> [w305 w311]
                          frame False {
                            n219 = Concatenate Strings(w305, "_" ("string"), w303, ".csv" ("string")) -> (w306:string)
                            n220 = Build Path(base path=w308, name or relative path=w306) -> (appended path=w307:path)
                          }
                          frame True {
                            n221 = Concatenate Strings(w311, "_m.csv" ("string")) -> (w310:string)
                            n222 = Build Path(base path=w312, name or relative path=w310) -> (appended path=w313:path)
                          }
                        }
                      }
                    }
                    n223 = case shown="False" w289 {
                      tunnel: w290 -> [w315 _]
                      tunnel: w288 -> [w314 _]
                      tunnel: w287 -> [_ _]
                      frame False {
                        n224 = call-poly <vilib>:"Write Delimited Spreadsheet.vi"("file path (dialog if empty)"=w314, "format (%.3f)"="%.9e", "2D data"=w315, "transpose? (no:F)"=TRUE, "delimiter (\\t)"="," ("delimiter (\\t)")) -> ()  [unwired: 9 in, 2 out]
                      }
                      frame True {
                      }
                    }
                  }
                }
                n225 = case shown="True" w271 {
                  tunnel: w278 -> [_ w327]
                  tunnel: w273 -> [_ w325]
                  tunnel: w269 -> [_ w324]
                  tunnel: w272 -> [_ w322]
                  tunnel: "Save Tag" -> [_ w320]
                  frame False {
                  }
                  frame True {
                    n226 = Concatenate Strings(w320, "|" ("string"), w324) -> (w321:string)
                    n227 = Search and Replace String(input string=w325, search string="JuncName" ("string"), replace string=w321) -> (result string=w326:string)  [unwired: 5 in, 3 out]
                    n228 = call "UploadIV.vi"("UiDefinition 2"=w322, "IV Scan Data"=w327, "url"=w326) -> ()  [unwired: 9 in]
                  }
                }
              }
            }
          }
          event "EnableJoystick": Value Change {
            n229 = event-data() -> ()  [unwired: 1 in, 6 out]
            n230 = case shown="True" "EnableJoystick" {
              frame False {
              }
              frame True {
                n231 = call "ReturnToJoystick.vi"() -> ()  [unwired: 12 in]
              }
            }
          }
          event "resetcontact": Value Change {
            n232 = event-data() -> ()  [unwired: 1 in, 6 out]
            n233 = case shown="True" "resetcontact" {
              tunnel: w330 -> [_ w335]
              frame False {
              }
              frame True {
                n234 = call "VXM_MotorPositionF.vi"() -> ("Position"=w344:i32[])  [unwired: 11 in]
                n235 = local write "In Contact"(FALSE ("In Contact")) -> ()
                n236 = Index Array(array=w344, index=2) -> (element=w342:i32)
                n237 = Add(x=-3000, y=w342) -> (x+y=w339:i32)
                n238 = call "StatusGood.vi"("Text.Text"="Please reset position 1") -> ()  [unwired: 11 in]
                n239 = Unbundle By Name(w335) -> ("ControlRefs.WaferAlignment"=w336:refnum<vi>)
                n240 = local read "Position 1"() -> (w340:i32[])
                n241 = property class="Clust (strict)"(reference=w336) -> ("Value"=w334:T1)  [unwired: 1 in, 2 out]
                n242 = Replace Array Subset(array=w340, new element=w339, index=2) -> (w333:i32[])
                n243 = local write "Position 1"(w333) -> ()
                n244 = Bundle By Name(cluster=w334, "Position 1"=w333) -> (w332:T1)
                n245 = local write "WaferAlignment"(w332) -> ()
              }
            }
          }
          event "Position 3": Value Change {
            # "Move to position 3"
            n246 = event-data() -> ()  [unwired: 1 in, 6 out]
            n247 = local read "In Contact"() -> (w349:bool)
            n248 = call "MovePos3.vi"("In Contact in"=w349, "Position 3"="Position 3", "UiDefinition 2"=w346) -> ("In Contact out"=w348:bool)  [unwired: 8 in]
            n249 = local write "In Contact"(w348) -> ()
          }
          event "Align Position 3": Value Change {
            n250 = event-data() -> ()  [unwired: 1 in, 6 out]
            n251 = case shown="True" "Align Position 3" {
              tunnel: w350 -> [_ w353]
              frame False {
              }
              frame True {
                n252 = call "VXM_MotorPositionF.vi"() -> ("Position"=w357:i32[])  [unwired: 11 in]
                "Position 3" <- w357
                n253 = control-ref of="Align Position 3"() -> (w360:refnum<vi>)
                n254 = property class="Bool"(reference=w360, "Colors [4]"=cluster{u32, u32}[] [{13816530, 13816530}]) -> ()  [unwired: 1 in, 2 out]
                n255 = Unbundle By Name(w353) -> ("ControlRefs.Status"=w352:refnum<vi>)
                n256 = Unbundle By Name(w353) -> ("ControlRefs.WaferAlignment"=w359:refnum<vi>)
                n257 = property class="Clust (strict)"(reference=w359) -> ("Value"=w358:T1)  [unwired: 1 in, 2 out]
                n258 = Bundle By Name(cluster=w358, "Position 3"=w357) -> (w354:T1)
                n259 = call "CheckAlignmentAngles.vi"("Status in"="Please return to position 1 and run cycle" ("Status"), "Value"=w354) -> ("Status out"=w355:string)  [unwired: 9 in]
                n260 = local write "WaferAlignment"(w354) -> ()
                n261 = call "StatusGood.vi"("Text.Text"=w355, "String in"=w352) -> ()  [unwired: 10 in]
              }
            }
          }
          event "ClearPositions": Value Change {
            n262 = event-data() -> ()  [unwired: 1 in, 6 out]
            n263 = case shown="True" "ClearPositions" {
              tunnel: w362 -> [_ w369]
              frame False {
              }
              frame True {
                w365 = cluster{u32, u32}[] [{16741120, 16741120}] ("Colors [4]")
                w364 = i32[] [] ("Position 3")
                n264 = control-ref of="Align Position 1"() -> (w366:refnum<vi>)
                n265 = control-ref of="Align Position 3"() -> (w370:refnum<vi>)
                n266 = property class="Bool"(reference=w370, "Colors [4]"=w365) -> ()  [unwired: 1 in, 2 out]
                n267 = control-ref of="Align Position 2"() -> (w367:refnum<vi>)
                n268 = Unbundle By Name(w369) -> ("ControlRefs.WaferAlignment"=w368:refnum<vi>)
                n269 = property class="Bool"(reference=w367, "Colors [4]"=w365) -> ()  [unwired: 1 in, 2 out]
                n270 = property class="Bool"(reference=w366, "Colors [4]"=w365) -> ()  [unwired: 1 in, 2 out]
                n271 = property class="Clust (strict)"(reference=w368) -> ("Value"=w372:T1)  [unwired: 1 in, 2 out]
                n272 = local write "Position 3"(w364) -> ()
                n273 = local write "Position 2"(w364) -> ()
                n274 = local write "Position 1"(w364) -> ()
                n275 = Bundle By Name(cluster=w372, "Position 3"=w364, "Position 1"=w364, "Position 2"=w364) -> (w371:T1)
                n276 = local write "WaferAlignment"(w371) -> ()
                n277 = call "StatusGood.vi"("Text.Text"="Please set position 1" ("Status")) -> ()  [unwired: 11 in]
              }
            }
          }
          event "Align Position 2": Value Change {
            # "Set Align to Position 2"
            n278 = event-data() -> ()  [unwired: 1 in, 6 out]
            n279 = Unbundle By Name(w375) -> ("ControlRefs.Status"=w374:refnum<vi>)
            n280 = case shown="True" "Align Position 2" {
              tunnel: w375 -> [_ w383]
              tunnel: w374 -> [_ w377]
              frame False {
              }
              frame True {
                n281 = Unbundle By Name(w383) -> ("Microsites"=w387:refnum<k24>)
                n282 = call "VXM_MotorPositionF.vi"() -> ("Position"=w384:i32[])  [unwired: 11 in]
                "Position 2" <- w384
                n283 = local read "Steps Per micron"() -> (w389:dbl)
                n284 = local read "Chip Orientation"() -> (w388:i32)
                n285 = control-ref of="Align Position 2"() -> (w390:refnum<vi>)
                n286 = local read "Position 1"() -> (w391:i32[])
                n287 = call "AlignPosition2.vi"("Chip Orientation"=w388, "Steps Per micron"=w389, "Position 1"=w391, "Microsites"=w387, "Boolean in"=w390) -> ("Array"=w381:dbl[], "Numeric"=w382:dbl)  [unwired: 5 in]
                n288 = Unbundle By Name(w383) -> ("ControlRefs.WaferAlignment"=w386:refnum<vi>)
                n289 = local write "Scale Misalign"(w382) -> ()
                n290 = local write "Rotation Misalign"(w381) -> ()
                n291 = property class="Clust (strict)"(reference=w386) -> ("Value"=w385:T1)  [unwired: 1 in, 2 out]
                n292 = Bundle By Name(cluster=w385, "Position 2"=w384, "Scale Misalign"=w382, "Rotation Misalign"=w381) -> (w378:T1)
                n293 = call "CheckAlignmentAngles.vi"("Status in"="Please return to position 1 and run cycle" ("Status"), "Value"=w378) -> ("Status out"=w379:string)  [unwired: 9 in]
                n294 = call "StatusGood.vi"("Text.Text"=w379, "String in"=w377) -> ()  [unwired: 10 in]
                n295 = local write "WaferAlignment"(w378) -> ()
              }
            }
          }
        }
        "UiDefinition 3" <- w182
      }
    }
    frame #6 {
      # "Close all tools"
      n296 = local read "VISA resource name"() -> (w393:refnum<visa-resource-name>)
      n297 = flat-sequence {
        frame #0 {
          n298 = call "Vxmdriverlv8.Vi"("Chars to send"="Q") -> ()  [unwired: 21 in, 6 out]
        }
        frame #1 {
          n299 = call "Vxmdriverlv8.Vi"("Close Port"=TRUE) -> ()  [unwired: 21 in, 6 out]
        }
      }
      n300 = call "Close.vi"("VISA resource name"=w393) -> ("error out"=w394:errorcluster)  [unwired: 10 in]
      n301 = call <vilib>:"Simple Error Handler.vi"("error in (no error)"=w394) -> ()  [unwired: 4 in, 5 out]
    }
  }
  n302 = case shown="True" w1 {
    frame False {
    }
    frame True {
      n303 = Stop(stop? (T)=TRUE) -> ()
    }
  }
